vi "DAQ_set_all.vi"(3 "Error In":errorcluster, 5 "DAQ Settings":T1={"Shutters Settings"=[{"Name"="Shutter 1", "DAQ Channel/line"="Dev1/port0/line0", "Active"=FALSE}, {"Name"="Shutter 2", "DAQ Channel/line"="Dev1/port0/line1", "Active"=FALSE}], "Shutter Task"="", "Acquire Settings"=[], "AI Task"="", "Sample mode"=10178, "Number of Samples"=0, "Rate"=0.0, "AI Name"="", "DO Name"=""} {"Sample mode" items=["Finite Samples"=10178, "Continuous Samples"=10123, "Hardware Timed Single Point"=12522]; "Acquire Settings"."input terminal configuration" items=["default"=-1, "RSE"=10083, "NRSE"=10078, "Differential"=10106, "Pseudodifferential"=12529]}) -> (0 "Error Out":errorcluster, 2 "DAQ Out":T1={"Shutters Settings"=[{"Name"="Shutter 1", "DAQ Channel/line"="Dev1/port0/line0", "Active"=FALSE}, {"Name"="Shutter 2", "DAQ Channel/line"="Dev1/port0/line1", "Active"=FALSE}], "Shutter Task"="", "Acquire Settings"=[], "AI Task"="", "Sample mode"=10178, "Number of Samples"=0, "Rate"=0.0, "AI Name"="", "DO Name"=""} {"Sample mode" items=["Finite Samples"=10178, "Continuous Samples"=10123, "Hardware Timed Single Point"=12522]; "Acquire Settings"."input terminal configuration" items=["default"=-1, "RSE"=10083, "NRSE"=10078, "Differential"=10106, "Pseudodifferential"=12529]})   [LabVIEW 2020]
uses:
  Type defs/DAQ_set_Ctrl.ctl
  Type defs/DAQ_Shutter_Ctrl.ctl
  Type defs/DAQ_AI_Ctrl.ctl
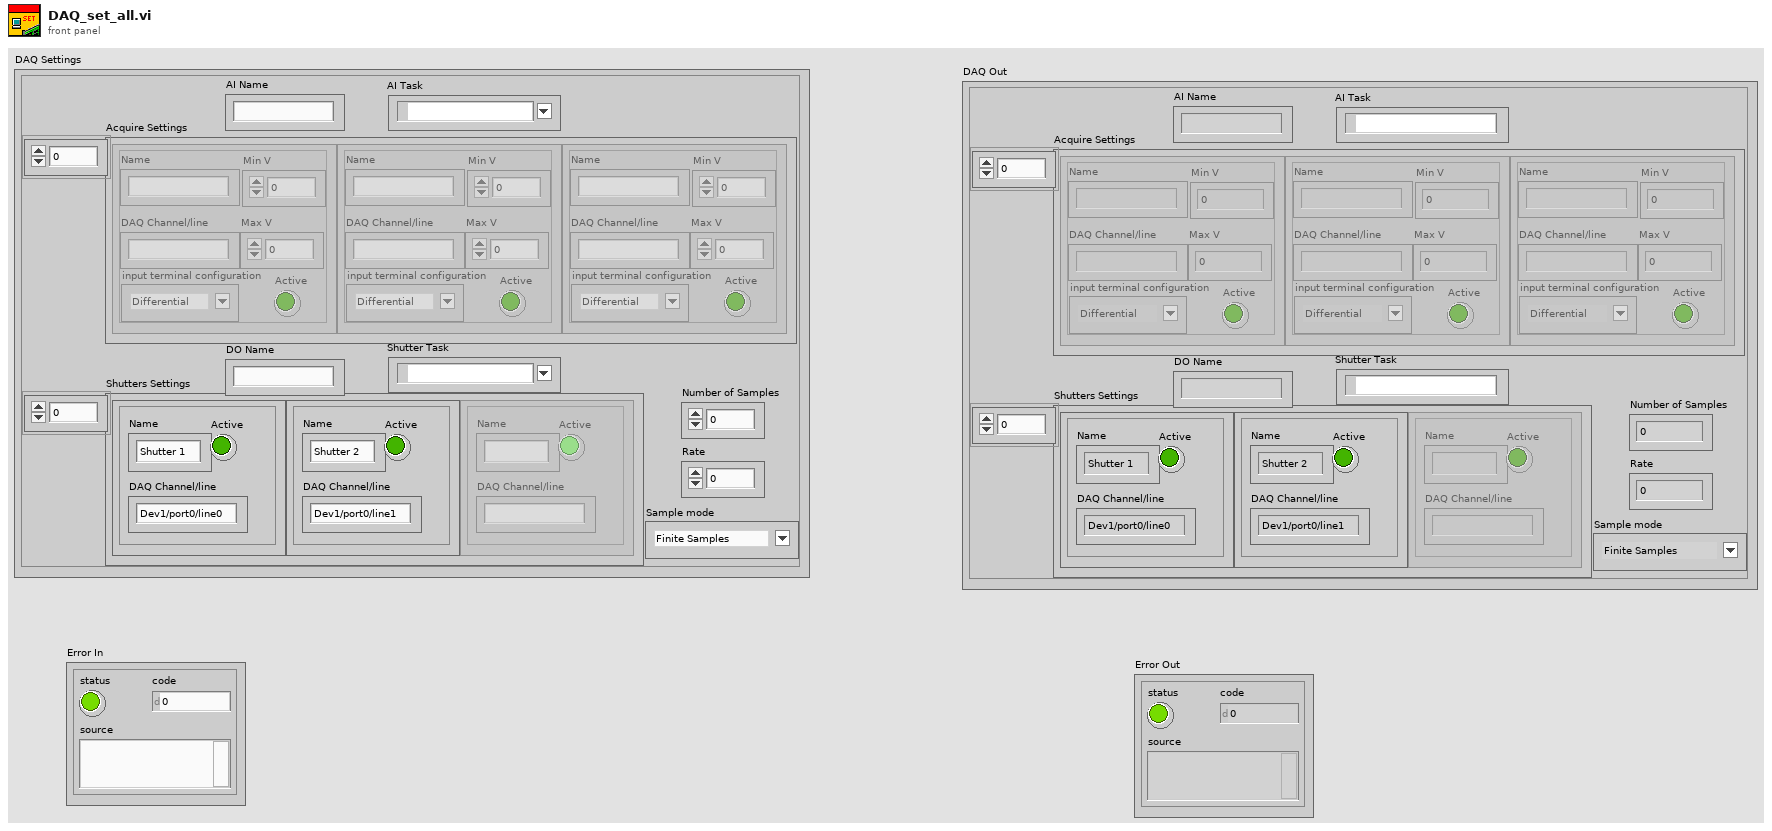
[diagram p1: front panel]
types:
  T1 = typedef "DAQ_set_Ctrl.ctl" = cluster{"Shutters Settings":T2[], "Shutter Task":refnum<k21>, "Acquire Settings":T3[], "AI Task":refnum<k21>, "Sample mode":i32, "Number of Samples":i32, "Rate":dbl, "AI Name":string, "DO Name":string}
  T2 = typedef "DAQ_Shutter_Ctrl.ctl" = cluster{"Name":string, "DAQ Channel/line":string, "Active":bool}
  T3 = typedef "DAQ_AI_Ctrl.ctl" = cluster{"Name":string, "DAQ Channel/line":string, "Max V":dbl, "Min V":dbl, "input terminal configuration":i32, "Active":bool}
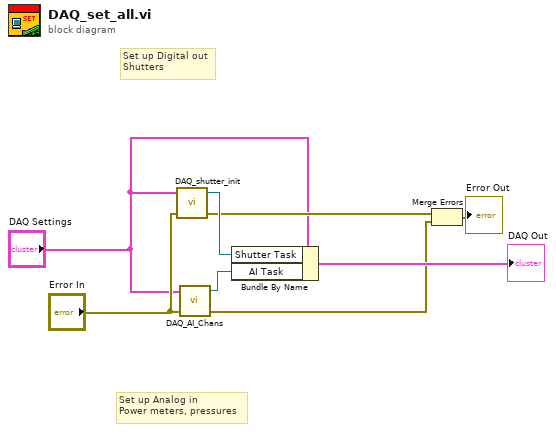
[diagram p0: block diagram]
diagram:
  # "Set up Analog in\nPower meters, pressures"
  # "Set up Digital out\nShutters"
  n1 = call "DAQ_shutter_init.vi"("error in"="Error In", "DAQ Settings"="DAQ Settings") -> ("error out"=w6:errorcluster, "DO Task"=w7:refnum<k21>)  [unwired: 2 in]
  n2 = call "DAQ_AI_Chans.vi"("error in"="Error In", "DAQ Settings"="DAQ Settings") -> ("error out"=w2:errorcluster, "Acquire Out"=w4:refnum<k21>)  [unwired: 2 in]
  n3 = Bundle By Name(cluster="DAQ Settings", "Shutter Task"=w7, "AI Task"=w4) -> (→"DAQ Out":T1)
  n4 = Merge Errors(w6, w2) -> (→"Error Out":errorcluster)
